vi "loader.vi"() -> ()   [LabVIEW 2013, in "configuration tests.lvlib"]
uses:
  configuration tests.lvlib
  <vilib>/NI/Tag Bus Module Framework/root configuration/TBM configuration.lvclass
  <vilib>/NI/Tag Bus Module Framework/module configuration/TBM module configuration.lvclass
  <vilib>/NI/Tag Bus Module Framework/channel/TBM channel.lvclass
  <vilib>/NI/Module Execution Interface/Engine Configuration/engine configuration.lvclass
  <vilib>/NI/Module Timing Source/timing source/TBM timing source.lvclass
  Framework Configuration Classes/system configuration/PL_System Configuration.lvclass
  <vilib>/NI/Configuration Framework/Repository/NISE_CEF_Repository.lvclass
  <vilib>/NI/Configuration Framework/Node/NISE_CEF_Node.lvclass
  Configuration Editor/Classes/TBM Configuration Node/TBM Configuration Node.lvclass
  Configuration Editor/Classes/Module editor node/module editor node.lvclass
  Configuration Editor/Classes/EngineTags/EngineTags.lvclass
  Configuration Editor/Classes/Engine Parent/Engine Parent Editor Node.lvclass
  Configuration Editor/Classes/Targets/Targets.lvclass
  Configuration Editor/Classes/Systems/Systems.lvclass
  Configuration Editor/Classes/SystemConfigRepo/SystemConfigRepo.lvclass
  Framework Configuration Classes/target configuration/PL_Target Configuration.lvclass
panel:
  out "Array 2":refnum<class>[](array[class])
  in  "stop":bool
  out "Array":errorcluster[](array[cluster])
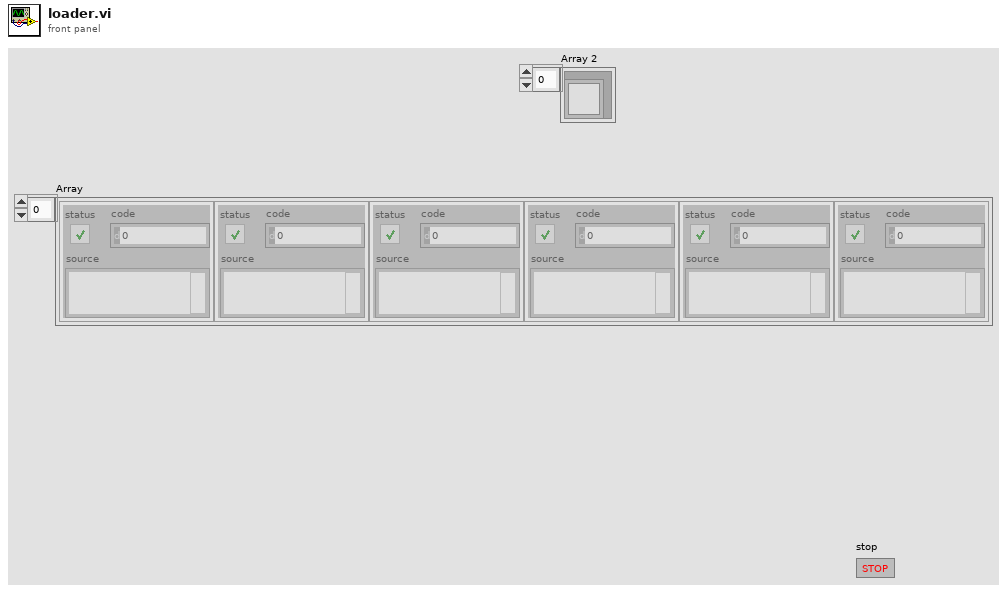
[diagram p1: front panel]
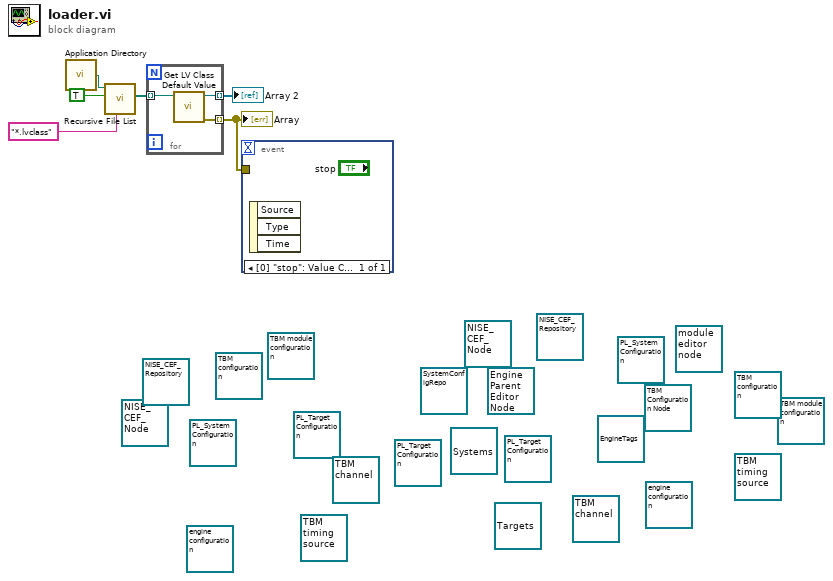
[diagram p0: block diagram]
diagram:
  (unwired) refnum<class "PL_Target Configuration.lvclass"> refnum ("Target Configuration")
  (unwired) refnum<class "SystemConfigRepo.lvclass"> refnum ("PL Framework Configuration Tool.lvlib:SystemConfigRepo.lvclass")
  (unwired) refnum<class "Systems.lvclass"> refnum ("PL Framework Configuration Tool.lvlib:Systems.lvclass")
  (unwired) refnum<class "Targets.lvclass"> refnum ("PL Framework Configuration Tool.lvlib:Targets")
  (unwired) refnum<class "Engine Parent Editor Node.lvclass"> refnum ("PL Framework Configuration Tool.lvlib:Engine Parent Editor Node.lvclass")
  (unwired) refnum<class "EngineTags.lvclass"> refnum ("PL Framework Configuration Tool.lvlib:EngineTags.lvclass")
  (unwired) refnum<class "module editor node.lvclass"> refnum ("PL Framework Configuration Tool.lvlib:module editor node.lvclass")
  (unwired) refnum<class "TBM Configuration Node.lvclass"> refnum ("PL Framework Configuration Tool.lvlib:TBM Configuration Node")
  (unwired) refnum<class "NISE_CEF_Node.lvclass"> refnum ("NISE_CEF_Node.lvclass")
  (unwired) refnum<class "NISE_CEF_Repository.lvclass"> refnum ("NISE_CEF_Repository.lvclass")
  (unwired) refnum<class "PL_Target Configuration.lvclass"> refnum ("Target Configuration")
  (unwired) refnum<class "PL_System Configuration.lvclass"> refnum ("System Configuration")
  (unwired) refnum<class "TBM timing source.lvclass"> refnum ("TBM timing source.lvclass")
  (unwired) refnum<class "engine configuration.lvclass"> refnum ("engine configuration.lvclass")
  (unwired) refnum<class "TBM channel.lvclass"> refnum ("channel")
  (unwired) refnum<class "TBM module configuration.lvclass"> refnum ("module configuration")
  (unwired) refnum<class "TBM configuration.lvclass"> refnum ("configuration")
  (unwired) refnum<class "NISE_CEF_Node.lvclass"> refnum ("NISE_CEF_Node.lvclass")
  (unwired) refnum<class "NISE_CEF_Repository.lvclass"> refnum ("NISE_CEF_Repository.lvclass")
  (unwired) refnum<class "PL_Target Configuration.lvclass"> refnum ("Target Configuration")
  (unwired) refnum<class "PL_System Configuration.lvclass"> refnum ("System Configuration")
  (unwired) refnum<class "TBM timing source.lvclass"> refnum ("TBM timing source.lvclass")
  (unwired) refnum<class "engine configuration.lvclass"> refnum ("engine configuration.lvclass")
  (unwired) refnum<class "TBM channel.lvclass"> refnum ("channel")
  (unwired) refnum<class "TBM module configuration.lvclass"> refnum ("module configuration")
  (unwired) refnum<class "TBM configuration.lvclass"> refnum ("configuration")
  n1 = call <vilib>:"Application Directory.vi"() -> ("Application Directory"=w6:path)
  n2 = call <vilib>:"Recursive File List.vi"("pattern"="*.lvclass", "Treat LLBs as Folders?"=TRUE, "Folder Path"=w6) -> ("All Files in Dir"=w3:path[])  [unwired: 4 in, 4 out]
  n3 = for {
    tunnel: w3 -> [w9] mode=indexing
    tunnel: [w8] -> w2 mode=indexing
    tunnel: [w7] -> w1 mode=indexing
    n4 = call <vilib>:"Get LV Class Default Value.vi"("class path"=w9) -> ("error out"=w8:errorcluster, "object"=w7:refnum<class>)  [unwired: 9 in]
  }
  "Array" <- w2
  "Array 2" <- w1
  n5 = event shown="[0] \"stop\": Value Change;  Application Instance Close;  Panel Close" {
    selector: _ -> [_]
    dyn-events: _ -> [_]
    timeout: _ -> [_]
    tunnel: w2 -> [_]
    event "stop": Value Change; Application Instance Close; Panel Close {
      n6 = event-data() -> ()  [unwired: 1 in, 3 out]
    }
  }
